vi "TransmitMIMICCommand.vi"(3 "Error In":errorcluster, 4 "CheckSum?":bool, 5 "Command array":u8[](array[numeric]) format="%x") -> (0 "Error Out":errorcluster, 1 "MIMIC_CMD":string, 2 "Status":bool)   [LabVIEW 2014]
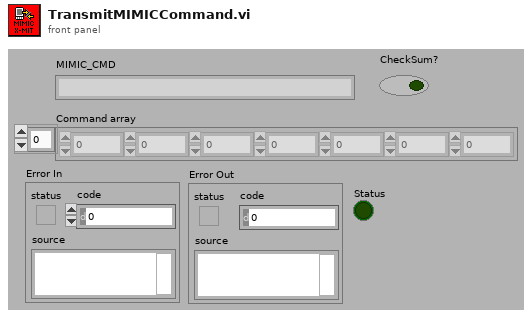
[diagram p1: front panel]
types:
  T1 = enum16{"OpenPort", "Initial Serial Port", "Write", "ByteRead", "Read", "ClearBuff", "Close"}
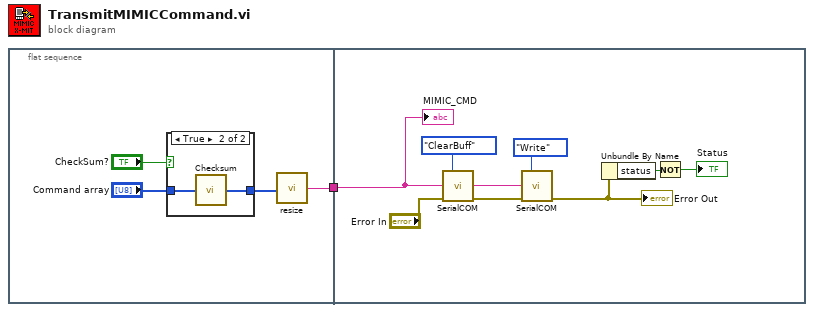
[diagram p0: block diagram]
diagram:
  n1 = flat-sequence {
    tunnel: [w2] -> w1
    tunnel: w1 -> [w9]
    frame #0 {
      n2 = case shown="True" "CheckSum?" {
        tunnel: "Command array" -> [w6 w8]
        tunnel: [w6 w7] -> w4
        frame False {
        }
        frame True {
          n3 = call "Checksum.vi"("INPUT_Array"=w8) -> ("OUTPUT_Array"=w7:u8[])
        }
      }
      n4 = call "resize.vi"("Array"=w4) -> ("MIMIC_CMD"=w2:string)
    }
    frame #1 {
      n5 = call "SerialCOM.vi"("Function"=T1."ClearBuff", "error in (no error)"="Error In") -> ("error out"=w14:errorcluster)  [unwired: 8 in, 5 out]
      n6 = call "SerialCOM.vi"("Function"=T1."Write", "write buffer"=w9, "error in (no error)"=w14) -> ("error out"=w12:errorcluster)  [unwired: 7 in, 5 out]
      "Error Out" <- w12
      n7 = Unbundle By Name(w12) -> ("status"=w11:bool)
      n8 = Not(x=w11) -> (.not. x?=→"Status":bool)
      "MIMIC_CMD" <- w9
    }
  }
